vi "generat.vi"(11 "Количество бит":i32) -> (3 "Array":dbl[](array[numeric]))   [LabVIEW 2017]
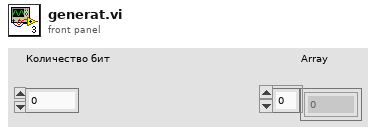
[diagram p1: front panel]
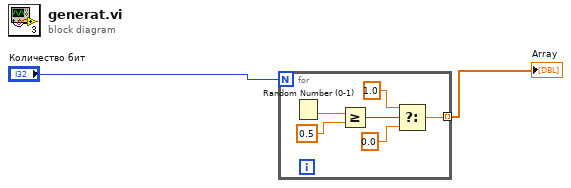
[diagram p0: block diagram]
diagram:
  n1 = for {
    N: "Количество бит" -> [_]
    tunnel: [w3] -> w2 mode=indexing
    n2 = Random Number (0-1)() -> (number: 0 to 1=w8:dbl)
    n3 = Greater Or Equal?(x=w8, y=0.5) -> (x >= y?=w6:bool)
    n4 = Select(t=1.0, s=w6, f=0.0) -> (s? t:f=w3:dbl)
  }
  "Array" <- w2
